vi "setSerializedData.vi"(0 "reference in":refnum<class "DQMHModuleNode.lvclass">, 1 "parent":refnum<class "AbstractNode.lvclass">, 2 "children":refnum<class "AbstractNode.lvclass">[](array[class]), 3 "xmlIn":string, 5 "error in (no error)":errorcluster) -> (14 "reference out":refnum<class "DQMHModuleNode.lvclass">, 19 "error out":errorcluster)   [LabVIEW 2014, in "DQMHModuleNode.lvclass"]
doc: "Sets stored data"
uses:
  <resource>/Framework/Providers/Open_GDS/UML/DQMHModuleNode_class/DQMHModuleNode.lvclass
  <resource>/Framework/Providers/Open_GDS/UML/AbstractNode_class/AbstractNode.lvclass
  <resource>/Framework/Providers/Open_GDS/UML/AbstractNode_class/protected/ObjectAttributes.ctl
  <resource>/Framework/Providers/Open_GDS/UML/RectangularNode_class/protected/ObjectAttributes.ctl
  <resource>/Framework/Providers/Open_GDS/UML/General/Rectangle/Rectangle Rectangle2D.ctl
  <resource>/Framework/Providers/Open_GDS/UML/DQMHModuleNode_class/protected/ObjectAttributes.ctl
  <resource>/Framework/Providers/Open_GDS/UML/MultiLineString_class/MultiLineString.lvclass
  <resource>/Framework/Providers/Open_GDS/UML/RectangularNode_class/RectangularNode.lvclass
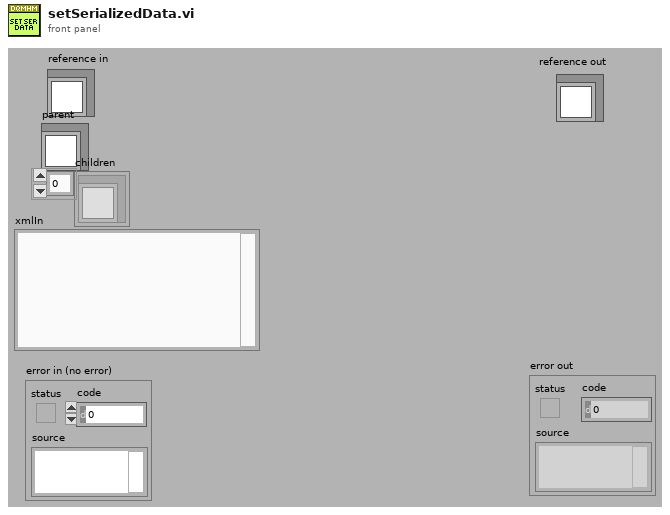
[diagram p1: front panel]
types:
  T1 = cluster{"data string":string, "text":string, "text":string, "text":string, "text":string}
  T2 = typedef "AbstractNode.lvclass/ObjectAttributes.ctl" = cluster{"parent":refnum<class "AbstractNode.lvclass">, "children":refnum<class "AbstractNode.lvclass">[], "Hidden":bool}
  T3 = typedef "RectangularNode.lvclass/ObjectAttributes.ctl" = cluster{"bounds":T4}
  T4 = typedef "Rectangle Rectangle2D.ctl" = cluster{"x":dbl, "y":dbl, "width":dbl, "height":dbl}
  T5 = typedef "DQMHModuleNode.lvclass/ObjectAttributes.ctl" = cluster{"midHeight":dbl, "botHeight":dbl, "Name":refnum<class "MultiLineString.lvclass">, "Description":refnum<class "MultiLineString.lvclass">, "InternalData":refnum<class "MultiLineString.lvclass">, "Events":refnum<class "MultiLineString.lvclass">, "DEFAULT_COMPARTMENT_HEIGHT":i32, "DEFAULT_WIDTH":i32, "DEFAULT_HEIGHT":i32, "showEvents":bool, "showInternalData":bool, "ClassPath":path, "Template":string, "Icon":u8[][]}
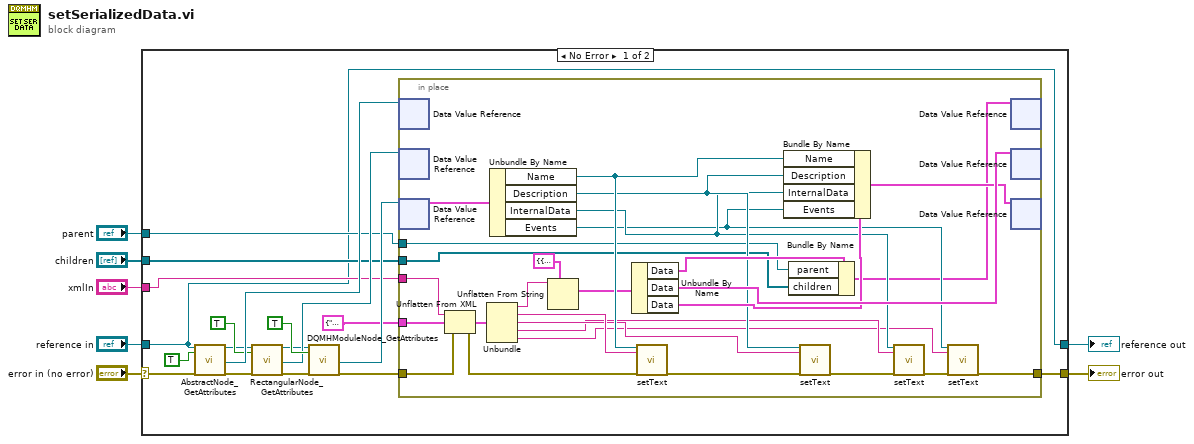
[diagram p0: block diagram]
diagram:
  n1 = case shown="No Error" "error in (no error)" {
    selector: "error in (no error)" -> [w16 w54]
    tunnel: "reference in" -> [w9 w55]
    tunnel: [w25 w54] -> w5
    tunnel: [w9 w55] -> w4
    tunnel: "xmlIn" -> [w20 _]
    tunnel: "parent" -> [w19 _]
    tunnel: "children" -> [w18 _]
    frame No Error {
      n2 = call <resource>:"AbstractNode_GetAttributes.vi"("reference in"=w9, "OnlyGetDvrReference(False)"=TRUE, "error in (no error)"=w16) -> ("reference out"=w13:refnum<class "DQMHModuleNode.lvclass">, "DataRef"=w21:refnum<data-value>, "error out"=w14:errorcluster)  [unwired: 13 in, 1 out]
      n3 = call <resource>:"RectangularNode_GetAttributes.vi"("reference in"=w13, "OnlyGetDvrReference(False)"=TRUE, "error in (no error)"=w14) -> ("reference out"=w12:refnum<class "DQMHModuleNode.lvclass">, "DataRef"=w22:refnum<data-value>, "error out"=w11:errorcluster)  [unwired: 13 in, 1 out]
      n4 = call <resource>:"DQMHModuleNode_GetAttributes.vi"("reference in"=w12, "OnlyGetDvrReference(False)"=TRUE, "error in (no error)"=w11) -> ("DataRef"=w23:refnum<data-value>, "error out"=w10:errorcluster)  [unwired: 13 in, 2 out]
      n5 = in-place {
        in-place-border: [w34] -> w25
        in-place-border: w10 -> [w30]
        in-place-border: T1 {"data string"="", "text"="", "text"="", "text"="", "text"=""} ("output cluster") -> [w52]
        in-place-border: w20 -> [w53]
        in-place-border: w19 -> [w32]
        in-place-border: w18 -> [w31]
        n6 = in-place-dvr #1(w21) -> ()  [unwired: 2 out]
        n7 = in-place-dvr #2(w22) -> ()  [unwired: 2 out]
        n8 = in-place-dvr #3(w23) -> (w46:T5)  [unwired: 1 out]
        n9 = Unflatten From XML(xml string=w53, type=w52, error in (no error)=w30) -> (value=w51:T1, error out=w29:errorcluster)
        n10 = Unbundle(w51) -> ("data string"=w28:string, "text"=w44:string, "text"=w41:string, "text"=w37:string, "text"=w35:string)
        n11 = Unbundle By Name(w46) -> ("Name"=w45:refnum<class "MultiLineString.lvclass">, "Description"=w42:refnum<class "MultiLineString.lvclass">, "InternalData"=w38:refnum<class "MultiLineString.lvclass">, "Events"=w36:refnum<class "MultiLineString.lvclass">)
        n12 = Unflatten From String(type=cluster{"Data":T2, "Data":T3, "Data":T5} {"Data"={"parent"=refnum, "children"=[], "Hidden"=FALSE}, "Data"={"bounds"={"x"=0.0, "y"=0.0, "width"=0.0, "height"=0.0}}, "Data"={"midHeight"=0.0, "botHeight"=0.0, "Name"=refnum, "Description"=refnum, "InternalData"=refnum, "Events"=refnum, "DEFAULT_COMPARTMENT_HEIGHT"=0, "DEFAULT_WIDTH"=0, "DEFAULT_HEIGHT"=0, "showEvents"=FALSE, "showInternalData"=FALSE, "ClassPath"=path "", "Template"="", "Icon"=[]}}, binary string=w28) -> (value=w26:cluster{"Data":T2, "Data":T3, "Data":T5})  [unwired: 3 in, 2 out]
        n13 = Unbundle By Name(w26) -> ("Data"=w50:T2, "Data"=w49:T3, "Data"=w48:T5)
        n14 = call-dynamic "setText.vi"("reference"=w45, "text"=w44, "error in (no error)"=w29) -> ("error out"=w43:errorcluster)  [unwired: 15 in, 1 out]
        n15 = Bundle By Name(cluster=w48, "Name"=w45, "Description"=w42, "InternalData"=w38, "Events"=w36) -> (w47:T5)
        n16 = Bundle By Name(cluster=w50, "parent"=w32, "children"=w31) -> (w33:T2)
        n17 = call-dynamic "setText.vi"("reference"=w42, "text"=w41, "error in (no error)"=w43) -> ("error out"=w40:errorcluster)  [unwired: 15 in, 1 out]
        n18 = call-dynamic "setText.vi"("reference"=w38, "text"=w37, "error in (no error)"=w40) -> ("error out"=w39:errorcluster)  [unwired: 15 in, 1 out]
        n19 = call-dynamic "setText.vi"("reference"=w36, "text"=w35, "error in (no error)"=w39) -> ("error out"=w34:errorcluster)  [unwired: 15 in, 1 out]
        n20 = in-place-dvr #1(w33) -> ()  [unwired: 2 out]
        n21 = in-place-dvr #2(w49) -> ()  [unwired: 2 out]
        n22 = in-place-dvr #3(w47) -> ()  [unwired: 2 out]
      }
    }
    frame Error {
    }
  }
  "reference out" <- w4
  "error out" <- w5
